vi "Get Registration.vi"(11 "Event Msg Type Strategy in":refnum<class "Event Msg Type Strategy.lvclass">) -> (2 "Registration":refnum<event-registration>)   [LabVIEW 2021, in "jettl.lvlib" / "Msg Type Strategy.lvlib" / "Event Msg Type Strategy.lvclass"]
uses:
  Event Msg Type Strategy.lvclass
  Msg Strategy/Msg Strategy.lvclass
  Event Msg Type Strategy.lvclass/Event Msg Type Strategy.ctl
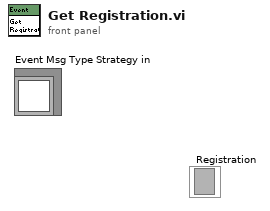
[diagram p1: front panel]
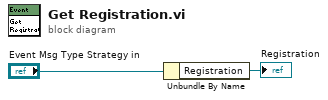
[diagram p0: block diagram]
diagram:
  n1 = Unbundle By Name("Event Msg Type Strategy in") -> ("Registration"=→"Registration":refnum<event-registration>)
